vi "Cycle_Diag_Table_Read.vi"(7 "ERD Data In":T3[](array[typedef]) {"ERD Number" format="%.0x"}, 11 "error in (no error)":errorcluster) -> (2 "Cycle Buffer Status":T2, 3 "Diag Cycle String Out":string[][](array[string]), 8 "Cycle  Diag Array Out":T1[](array[typedef]), 15 "error out":errorcluster)   [LabVIEW 2016]
uses:
  Common/LabVIEW GEA2 Toolkit/LabVIEW_GEA2_Toolkit.lvlibp/type defs/ERD Read Data Out.ctl
  type defs/Cycle_Diag_Buffer_Status.ctl
  type defs/Cycle_Diag.ctl
  Common/LabVIEW GEA2 Toolkit/LabVIEW_GEA2_Toolkit.lvlibp
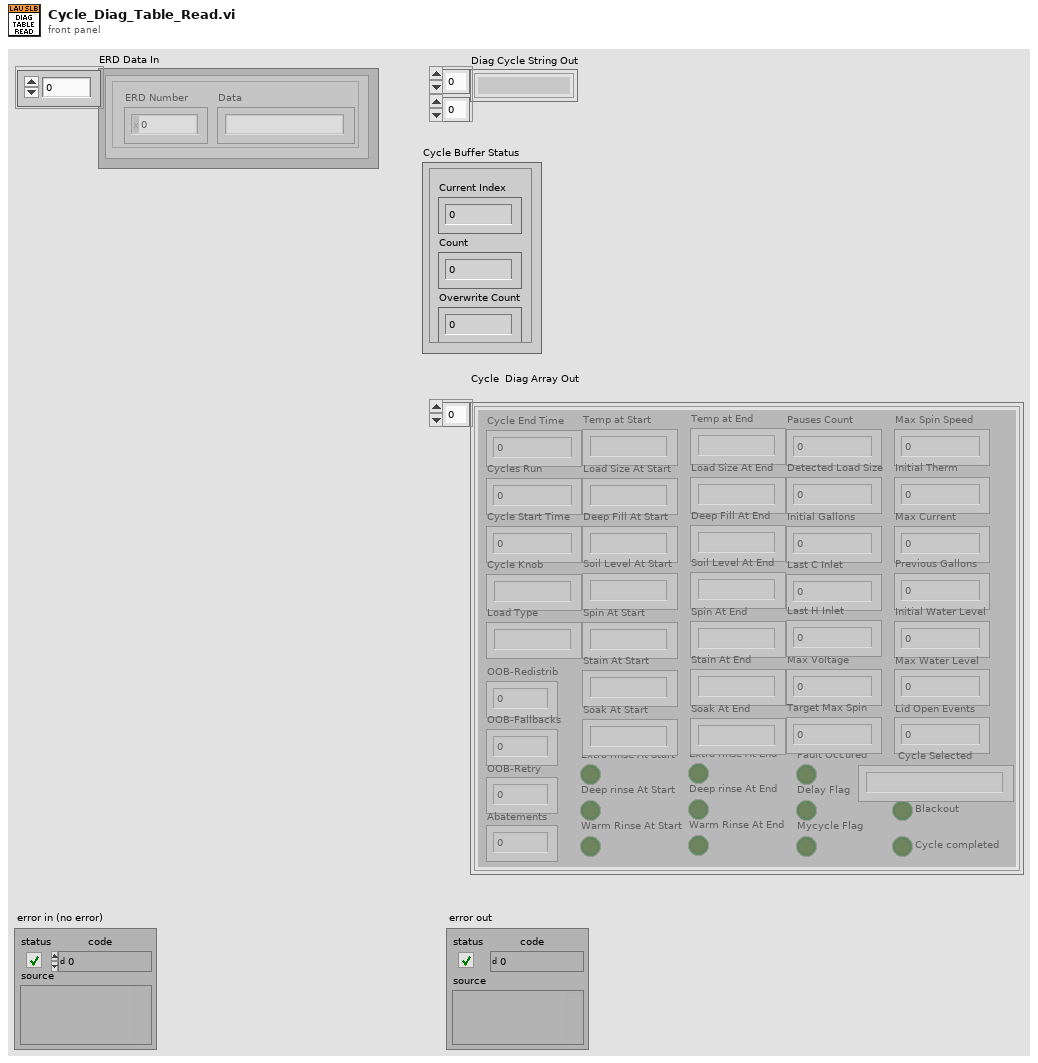
[diagram p1: front panel]
types:
  T1 = typedef "Cycle_Diag.ctl" = cluster{"Cycle End Time":u32, "Cycles Run":u32, "Cycle Start Time":u32, "Cycle Knob":string, "Load Type":string, "OOB-Redistrib":u8, "OOB-Fallbacks":u8, "OOB-Retry":u8, "Temp at Start":string, "Load Size At Start":string, "Deep Fill At Start":string, "Soil Level At Start":string, "Spin At Start":string, "Extra rinse At Start":bool, "Deep rinse At Start":bool, "Stain At Start":string, "Soak At Start":string, "Warm Rinse At Start":bool, "Temp at End":string, "Load Size At End":string, "Deep Fill At End":string, "Soil Level At End":string, "Spin At End":string, "Extra rinse At End":bool, "Deep rinse At End":bool, "Stain At End":string, "Soak At End":string, "Warm Rinse At End":bool, "Pauses Count":u8, "Fault Occured":bool, "Delay Flag":bool, "Mycycle Flag":bool, "Blackout":bool, "Cycle completed":bool, "Detected Load Size":dbl, "Initial Gallons":dbl, "Last C Inlet ":dbl, "Max Voltage":dbl, "Target Max Spin":u16, "Max Spin Speed":u16, "Initial Therm":dbl, "Max Current":dbl, "Previous Gallons":dbl, "Initial Water Level":dbl, "Max Water Level":dbl, "Abatements ":u8, "Lid Open Events":u8, "Cycle Selected":string, "Last H Inlet ":dbl}
  T2 = typedef "Cycle_Diag_Buffer_Status.ctl" = cluster{"Current Index":u16, "Count":u16, "Overwrite Count":u16}
  T3 = typedef "LabVIEW_GEA2_Toolkit.lvlibp/ERD Read Data Out.ctl" = cluster{"ERD Number":u16, "Data":string}
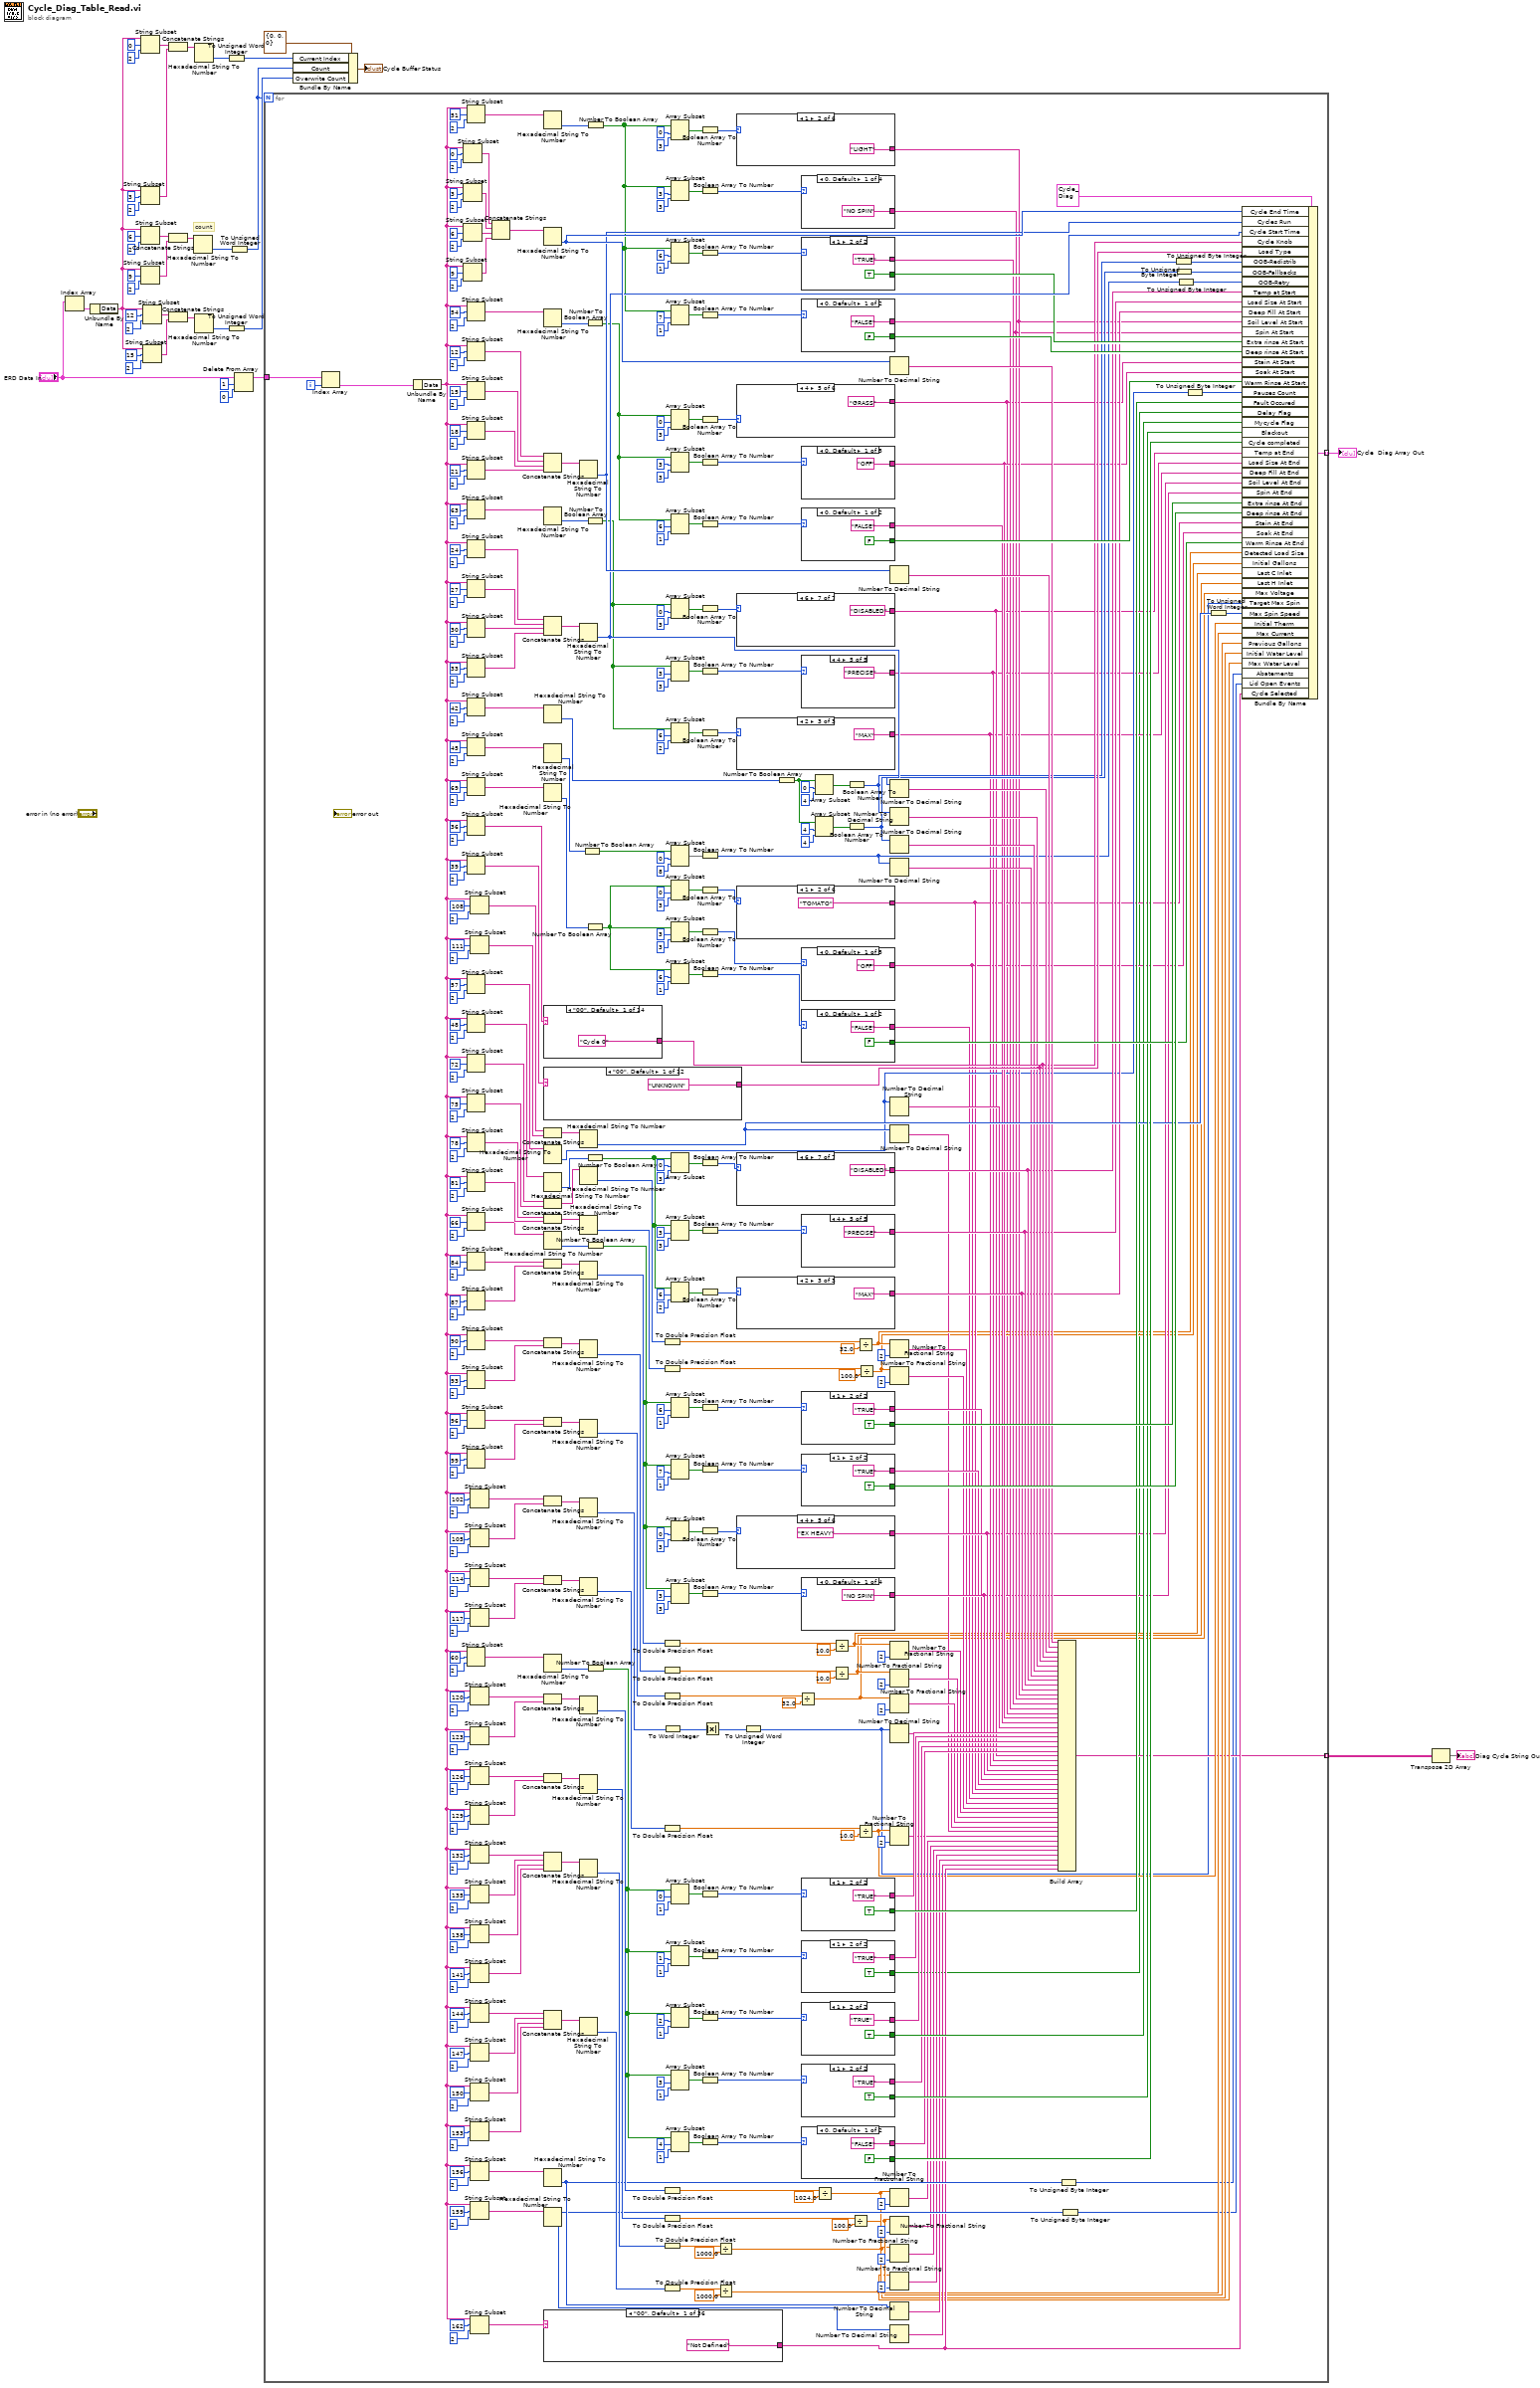
[diagram p0: block diagram]
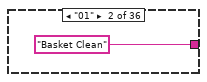
[diagram p2: hidden frame]
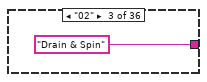
[diagram p3: hidden frame]
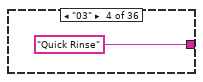
[diagram p4: hidden frame]
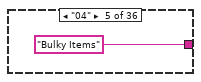
[diagram p5: hidden frame]
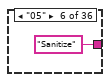
[diagram p6: hidden frame]
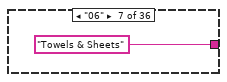
[diagram p7: hidden frame]
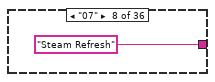
[diagram p8: hidden frame]
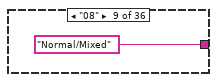
[diagram p9: hidden frame]
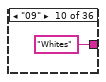
[diagram p10: hidden frame]
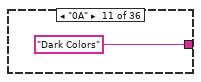
[diagram p11: hidden frame]
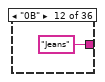
[diagram p12: hidden frame]
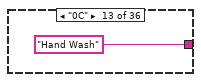
[diagram p13: hidden frame]
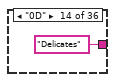
[diagram p14: hidden frame]
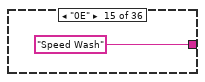
[diagram p15: hidden frame]
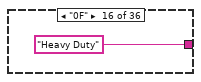
[diagram p16: hidden frame]
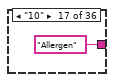
[diagram p17: hidden frame]
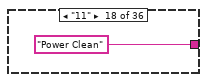
[diagram p18: hidden frame]
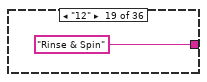
[diagram p19: hidden frame]
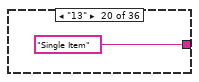
[diagram p20: hidden frame]
diagram:
  # "count"
  n1 = Index Array(array="ERD Data In") -> (element=w31:T3)  [unwired: 1 in]
  n2 = Unbundle By Name(w31) -> ("Data"=w11:string)
  n3 = String Subset(string=w11, offset (0)=0, length (rest)=2 ("length (rest)")) -> (substring=w20:string)
  n4 = String Subset(string=w11, offset (0)=3, length (rest)=2 ("length (rest)")) -> (substring=w21:string)
  n5 = String Subset(string=w11, offset (0)=6, length (rest)=2 ("length (rest)")) -> (substring=w35:string)
  n6 = String Subset(string=w11, offset (0)=9, length (rest)=2 ("length (rest)")) -> (substring=w34:string)
  n7 = String Subset(string=w11, offset (0)=12, length (rest)=2 ("length (rest)")) -> (substring=w22:string)
  n8 = String Subset(string=w11, offset (0)=15, length (rest)=2 ("length (rest)")) -> (substring=w23:string)
  n9 = Concatenate Strings(w20, w21) -> (w24:string)
  n10 = Concatenate Strings(w35, w34) -> (w33:string)
  n11 = Concatenate Strings(w22, w23) -> (w25:string)
  n12 = Hexadecimal String To Number(string=w33) -> (number=w32:u32)  [unwired: 2 in, 1 out]
  n13 = Hexadecimal String To Number(string=w24) -> (number=w26:u32)  [unwired: 2 in, 1 out]
  n14 = Hexadecimal String To Number(string=w25) -> (number=w27:u32)  [unwired: 2 in, 1 out]
  n15 = To Unsigned Word Integer(number=w26) -> (unsigned 16bit integer=w28:u16)
  n16 = To Unsigned Word Integer(number=w27) -> (unsigned 16bit integer=w29:u16)
  n17 = To Unsigned Word Integer(number=w32) -> (unsigned 16bit integer=w10:u16)
  n18 = Delete From Array(array="ERD Data In", length=1, index=0) -> (array with subset deleted=w7:T3[])  [unwired: 1 out]
  n19 = for {
    N: w10 -> [_]
    tunnel: w7 -> [w237]
    tunnel: [w233] -> w3 mode=indexing
    tunnel: [w170] -> w2 mode=indexing
    i -> [w236]
    n20 = Index Array(array=w237, index=w236) -> (element=w235:T3)
    n21 = Unbundle By Name(w235) -> ("Data"=w234:string)
    n22 = String Subset(string=w234, offset (0)=0, length (rest)=2 ("length (rest)")) -> (substring=w451:string)
    n23 = String Subset(string=w234, offset (0)=3, length (rest)=2 ("length (rest)")) -> (substring=w450:string)
    n24 = String Subset(string=w234, offset (0)=6, length (rest)=2 ("length (rest)")) -> (substring=w449:string)
    n25 = String Subset(string=w234, offset (0)=9, length (rest)=2 ("length (rest)")) -> (substring=w448:string)
    n26 = String Subset(string=w234, offset (0)=51, length (rest)=2 ("length (rest)")) -> (substring=w148:string)
    n27 = String Subset(string=w234, offset (0)=54, length (rest)=2 ("length (rest)")) -> (substring=w132:string)
    n28 = String Subset(string=w234, offset (0)=12, length (rest)=2 ("length (rest)")) -> (substring=w445:string)
    n29 = String Subset(string=w234, offset (0)=15, length (rest)=2 ("length (rest)")) -> (substring=w444:string)
    n30 = String Subset(string=w234, offset (0)=18, length (rest)=2 ("length (rest)")) -> (substring=w443:string)
    n31 = String Subset(string=w234, offset (0)=21, length (rest)=2 ("length (rest)")) -> (substring=w442:string)
    n32 = String Subset(string=w234, offset (0)=63, length (rest)=2 ("length (rest)")) -> (substring=w119:string)
    n33 = String Subset(string=w234, offset (0)=24, length (rest)=2 ("length (rest)")) -> (substring=w439:string)
    n34 = String Subset(string=w234, offset (0)=27, length (rest)=2 ("length (rest)")) -> (substring=w438:string)
    n35 = String Subset(string=w234, offset (0)=30, length (rest)=2 ("length (rest)")) -> (substring=w437:string)
    n36 = String Subset(string=w234, offset (0)=33, length (rest)=2 ("length (rest)")) -> (substring=w436:string)
    n37 = String Subset(string=w234, offset (0)=42, length (rest)=2 ("length (rest)")) -> (substring=w88:string)
    n38 = String Subset(string=w234, offset (0)=45, length (rest)=2 ("length (rest)")) -> (substring=w79:string)
    n39 = String Subset(string=w234, offset (0)=69, length (rest)=2 ("length (rest)")) -> (substring=w92:string)
    n40 = String Subset(string=w234, offset (0)=36, length (rest)=2 ("length (rest)")) -> (substring=w433:string)
    n41 = String Subset(string=w234, offset (0)=39, length (rest)=2 ("length (rest)")) -> (substring=w432:string)
    n42 = String Subset(string=w234, offset (0)=57, length (rest)=2 ("length (rest)")) -> (substring=w390:string)
    n43 = String Subset(string=w234, offset (0)=48, length (rest)=2 ("length (rest)")) -> (substring=w167:string)
    n44 = String Subset(string=w234, offset (0)=72, length (rest)=2 ("length (rest)")) -> (substring=w374:string)
    n45 = String Subset(string=w234, offset (0)=75 ("offset"), length (rest)=u32 2 ("default (0 U32)")) -> (substring=w371:string)
    n46 = String Subset(string=w234, offset (0)=78, length (rest)=2 ("length (rest)")) -> (substring=w366:string)
    n47 = String Subset(string=w234, offset (0)=81, length (rest)=2 ("length (rest)")) -> (substring=w365:string)
    n48 = String Subset(string=w234, offset (0)=66, length (rest)=2 ("length (rest)")) -> (substring=w105:string)
    n49 = String Subset(string=w234, offset (0)=84, length (rest)=2 ("length (rest)")) -> (substring=w355:string)
    n50 = String Subset(string=w234, offset (0)=87, length (rest)=2 ("length (rest)")) -> (substring=w354:string)
    n51 = String Subset(string=w234, offset (0)=90, length (rest)=2 ("length (rest)")) -> (substring=w349:string)
    n52 = String Subset(string=w234, offset (0)=93, length (rest)=2 ("length (rest)")) -> (substring=w348:string)
    n53 = String Subset(string=w234, offset (0)=96, length (rest)=2 ("length (rest)")) -> (substring=w339:string)
    n54 = String Subset(string=w234, offset (0)=99, length (rest)=2 ("length (rest)")) -> (substring=w338:string)
    n55 = String Subset(string=w234, offset (0)=60, length (rest)=2 ("length (rest)")) -> (substring=w389:string)
    n56 = String Subset(string=w234, offset (0)=108, length (rest)=2 ("length (rest)")) -> (substring=w326:string)
    n57 = String Subset(string=w234, offset (0)=111, length (rest)=2 ("length (rest)")) -> (substring=w325:string)
    n58 = String Subset(string=w234, offset (0)=102, length (rest)=2 ("length (rest)")) -> (substring=w329:string)
    n59 = String Subset(string=w234, offset (0)=105, length (rest)=2 ("length (rest)")) -> (substring=w328:string)
    n60 = String Subset(string=w234, offset (0)=114, length (rest)=2 ("length (rest)")) -> (substring=w314:string)
    n61 = String Subset(string=w234, offset (0)=117, length (rest)=2 ("length (rest)")) -> (substring=w313:string)
    n62 = String Subset(string=w234, offset (0)=120, length (rest)=2 ("length (rest)")) -> (substring=w304:string)
    n63 = String Subset(string=w234, offset (0)=123, length (rest)=2 ("length (rest)")) -> (substring=w303:string)
    n64 = String Subset(string=w234, offset (0)=126, length (rest)=2 ("length (rest)")) -> (substring=w294:string)
    n65 = String Subset(string=w234, offset (0)=129, length (rest)=2 ("length (rest)")) -> (substring=w293:string)
    n66 = String Subset(string=w234, offset (0)=132, length (rest)=2 ("length (rest)")) -> (substring=w284:string)
    n67 = String Subset(string=w234, offset (0)=135, length (rest)=2 ("length (rest)")) -> (substring=w283:string)
    n68 = String Subset(string=w234, offset (0)=138, length (rest)=2 ("length (rest)")) -> (substring=w253:string)
    n69 = String Subset(string=w234, offset (0)=141, length (rest)=2 ("length (rest)")) -> (substring=w252:string)
    n70 = String Subset(string=w234, offset (0)=144, length (rest)=2 ("length (rest)")) -> (substring=w278:string)
    n71 = String Subset(string=w234, offset (0)=147, length (rest)=2 ("length (rest)")) -> (substring=w277:string)
    n72 = String Subset(string=w234, offset (0)=150, length (rest)=2 ("length (rest)")) -> (substring=w247:string)
    n73 = String Subset(string=w234, offset (0)=153, length (rest)=2 ("length (rest)")) -> (substring=w246:string)
    n74 = String Subset(string=w234, offset (0)=156, length (rest)=2 ("length (rest)")) -> (substring=w258:string)
    n75 = String Subset(string=w234, offset (0)=159, length (rest)=2 ("length (rest)")) -> (substring=w257:string)
    n76 = String Subset(string=w234, offset (0)=162, length (rest)=2 ("length (rest)")) -> (substring=w254:string)
    n77 = Concatenate Strings(w451, w450, w449, w448) -> (w447:string)
    n78 = Hexadecimal String To Number(string=w148) -> (number=w155:u32)  [unwired: 2 in, 1 out]
    n79 = Hexadecimal String To Number(string=w447) -> (number=w446:u32)  [unwired: 2 in, 1 out]
    n80 = Hexadecimal String To Number(string=w132) -> (number=w140:u32)  [unwired: 2 in, 1 out]
    n81 = Concatenate Strings(w445, w444, w443, w442) -> (w441:string)
    n82 = Hexadecimal String To Number(string=w119) -> (number=w127:u32)  [unwired: 2 in, 1 out]
    n83 = Concatenate Strings(w439, w438, w437, w436) -> (w435:string)
    n84 = Hexadecimal String To Number(string=w88) -> (number=w87:u32)  [unwired: 2 in, 1 out]
    n85 = Hexadecimal String To Number(string=w79) -> (number=w78:u32)  [unwired: 2 in, 1 out]
    n86 = Hexadecimal String To Number(string=w92) -> (number=w100:u32)  [unwired: 2 in, 1 out]
    n87 = case shown="\"00\", Default" w433 {
      tunnel: ["Cycle 0" "Cycle 1" "Cycle 2" "Cycle 3" "Cycle 4" "Cycle 5" "Cycle 6" "Cycle 7" "Cycle 8" "Cycle 9" "Cycle 10" "Cycle 11" "Cycle 12" "Cycle 13"] -> w229
      frame "00", Default {
      }
      frame "01" {
      }
      frame "02" {
      }
      frame "03" {
      }
      frame "04" {
      }
      frame "05" {
      }
      frame "06" {
      }
      frame "07" {
      }
      frame "08" {
      }
      frame "09" {
      }
      frame "0A" {
      }
      frame "0B" {
      }
      frame "0C" {
      }
      frame "0D" {
      }
    }
    n88 = case shown="\"00\", Default" w432 {
      tunnel: ["UNKNOWN" "COTTON" "SYNTHETIC" "MIXED" "WET" "LOW FLOW" "SMALL" "MEDIUM" "LARGE" "SUPER" "SUPER PLUS" "MAX"] -> w228
      frame "00", Default {
      }
      frame "01" {
      }
      frame "02" {
      }
      frame "03" {
      }
      frame "04" {
      }
      frame "05" {
      }
      frame "06" {
      }
      frame "07" {
      }
      frame "08" {
      }
      frame "09" {
      }
      frame "0A" {
      }
      frame "0B" {
      }
    }
    n89 = Concatenate Strings(w326, w325) -> (w324:string)
    n90 = Hexadecimal String To Number(string=w390) -> (number=w212:u32)  [unwired: 2 in, 1 out]
    n91 = Hexadecimal String To Number(string=w167) -> (number=w166:u32)  [unwired: 2 in, 1 out]
    n92 = Concatenate Strings(w374, w371) -> (w370:string)
    n93 = Concatenate Strings(w366, w365) -> (w364:string)
    n94 = Hexadecimal String To Number(string=w105) -> (number=w115:u32)  [unwired: 2 in, 1 out]
    n95 = Concatenate Strings(w355, w354) -> (w353:string)
    n96 = Concatenate Strings(w349, w348) -> (w347:string)
    n97 = Concatenate Strings(w339, w338) -> (w337:string)
    n98 = Concatenate Strings(w329, w328) -> (w327:string)
    n99 = Concatenate Strings(w314, w313) -> (w312:string)
    n100 = Hexadecimal String To Number(string=w389) -> (number=w388:u32)  [unwired: 2 in, 1 out]
    n101 = Concatenate Strings(w304, w303) -> (w302:string)
    n102 = Concatenate Strings(w294, w293) -> (w292:string)
    n103 = Concatenate Strings(w284, w283, w253, w252) -> (w282:string)
    n104 = Concatenate Strings(w278, w277, w247, w246) -> (w276:string)
    n105 = Hexadecimal String To Number(string=w258) -> (number=w256:u32)  [unwired: 2 in, 1 out]
    n106 = Hexadecimal String To Number(string=w257) -> (number=w255:u32)  [unwired: 2 in, 1 out]
    n107 = case shown="\"00\", Default" w254 {
      tunnel: ["Not Defined" "Basket Clean" "Drain & Spin" "Quick Rinse" "Bulky Items" "Sanitize" "Towels & Sheets" "Steam Refresh" "Normal/Mixed" "Whites" "Dark Colors" "Jeans" "Hand Wash" "Delicates" "Speed Wash" "Heavy Duty" "Allergen" "Power Clean" "Rinse & Spin" "Single Item" "Colors" "Cold Wash" "Cottons" "Easy Care" "Active Wear" "Timed Dry" "Dewrinkle" "Air Fluff" "Steam Refresh" "Steam Dewrinkle" "Speed Dry" "Mixed" "Quick Dry" "Casuals" "Warm Up" "Energy Saver"] -> w179
      frame "00", Default {
      }
      frame "01" {
      }
      frame "02" {
      }
      frame "03" {
      }
      frame "04" {
      }
      frame "05" {
      }
      frame "06" {
      }
      frame "07" {
      }
      frame "08" {
      }
      frame "09" {
      }
      frame "0A" {
      }
      frame "0B" {
      }
      frame "0C" {
      }
      frame "0D" {
      }
      frame "0E" {
      }
      frame "0F" {
      }
      frame "10" {
      }
      frame "11" {
      }
      frame "12" {
      }
      frame "13" {
      }
      frame "14" {
      }
      frame "15" {
      }
      frame "80" {
      }
      frame "81" {
      }
      frame "82" {
      }
      frame "83" {
      }
      frame "84" {
      }
      frame "85" {
      }
      frame "86" {
      }
      frame "87" {
      }
      frame "88" {
      }
      frame "89" {
      }
      frame "8A" {
      }
      frame "8B" {
      }
      frame "8C" {
      }
      frame "8D" {
      }
    }
    n108 = Hexadecimal String To Number(string=w441) -> (number=w440:u32)  [unwired: 2 in, 1 out]
    n109 = Hexadecimal String To Number(string=w435) -> (number=w434:u32)  [unwired: 2 in, 1 out]
    n110 = Hexadecimal String To Number(string=w324) -> (number=w323:u32)  [unwired: 2 in, 1 out]
    n111 = Hexadecimal String To Number(string=w370) -> (number=w377:u32)  [unwired: 2 in, 1 out]
    n112 = Hexadecimal String To Number(string=w364) -> (number=w363:u32)  [unwired: 2 in, 1 out]
    n113 = Hexadecimal String To Number(string=w353) -> (number=w352:u32)  [unwired: 2 in, 1 out]
    n114 = Hexadecimal String To Number(string=w347) -> (number=w346:u32)  [unwired: 2 in, 1 out]
    n115 = Hexadecimal String To Number(string=w337) -> (number=w336:u32)  [unwired: 2 in, 1 out]
    n116 = Hexadecimal String To Number(string=w327) -> (number=w239:u32)  [unwired: 2 in, 1 out]
    n117 = Hexadecimal String To Number(string=w312) -> (number=w311:u32)  [unwired: 2 in, 1 out]
    n118 = Hexadecimal String To Number(string=w302) -> (number=w301:u32)  [unwired: 2 in, 1 out]
    n119 = Hexadecimal String To Number(string=w292) -> (number=w291:u32)  [unwired: 2 in, 1 out]
    n120 = Hexadecimal String To Number(string=w282) -> (number=w281:u32)  [unwired: 2 in, 1 out]
    n121 = Hexadecimal String To Number(string=w276) -> (number=w275:u32)  [unwired: 2 in, 1 out]
    n122 = Number To Boolean Array(number=w78) -> (Boolean array=w77:bool[])
    n123 = Number To Boolean Array(number=w140) -> (Boolean array=w139:bool[])
    n124 = Number To Boolean Array(number=w127) -> (Boolean array=w126:bool[])
    n125 = Number To Boolean Array(number=w100) -> (Boolean array=w99:bool[])
    n126 = Number To Boolean Array(number=w166) -> (Boolean array=w165:bool[])
    n127 = Number To Boolean Array(number=w155) -> (Boolean array=w147:bool[])
    n128 = Number To Boolean Array(number=w115) -> (Boolean array=w108:bool[])
    n129 = Number To Boolean Array(number=w388) -> (Boolean array=w63:bool[])
    n130 = To Double Precision Float(number=w377) -> (double precision float=w376:dbl)
    n131 = To Double Precision Float(number=w363) -> (double precision float=w362:dbl)
    n132 = To Double Precision Float(number=w352) -> (double precision float=w351:dbl)
    n133 = To Double Precision Float(number=w346) -> (double precision float=w345:dbl)
    n134 = To Double Precision Float(number=w336) -> (double precision float=w335:dbl)
    n135 = To Word Integer(number=w239) -> (16bit integer=w241:i16)
    n136 = To Double Precision Float(number=w311) -> (double precision float=w310:dbl)
    n137 = To Double Precision Float(number=w301) -> (double precision float=w300:dbl)
    n138 = To Double Precision Float(number=w291) -> (double precision float=w290:dbl)
    n139 = To Double Precision Float(number=w281) -> (double precision float=w280:dbl)
    n140 = To Double Precision Float(number=w275) -> (double precision float=w274:dbl)
    n141 = Array Subset(array=w147, index=0, length=3) -> (w144:bool[])
    n142 = Array Subset(array=w147, index=3, length=3) -> (w143:bool[])
    n143 = Array Subset(array=w147, index=6, length=1) -> (w142:bool[])
    n144 = Array Subset(array=w147, index=7, length=1) -> (w141:bool[])
    n145 = Array Subset(array=w139, index=0, length=3) -> (w130:bool[])
    n146 = Array Subset(array=w139, index=3, length=3) -> (w129:bool[])
    n147 = Array Subset(array=w139, index=6, length=1) -> (w128:bool[])
    n148 = Array Subset(array=w126, index=0, length=3) -> (w118:bool[])
    n149 = Array Subset(array=w126, index=3, length=3) -> (w117:bool[])
    n150 = Array Subset(array=w126, index=6, length=2) -> (w116:bool[])
    n151 = Array Subset(array=w77, index=0, length=8) -> (w74:bool[])
    n152 = Array Subset(array=w99, index=0, length=3) -> (w91:bool[])
    n153 = Array Subset(array=w99, index=3, length=3) -> (w90:bool[])
    n154 = Array Subset(array=w99, index=6, length=1) -> (w89:bool[])
    n155 = Array Subset(array=w165, index=0, length=3) -> (w158:bool[])
    n156 = Array Subset(array=w165, index=3, length=3) -> (w157:bool[])
    n157 = Array Subset(array=w165, index=6, length=2) -> (w156:bool[])
    n158 = Array Subset(array=w108, index=6, length=1) -> (w102:bool[])
    n159 = Array Subset(array=w108, index=7, length=1) -> (w101:bool[])
    n160 = Array Subset(array=w108, index=0, length=3) -> (w104:bool[])
    n161 = Array Subset(array=w108, index=3, length=3) -> (w103:bool[])
    n162 = Array Subset(array=w63, index=0, length=1) -> (w62:bool[])
    n163 = Array Subset(array=w63, index=1, length=1) -> (w60:bool[])
    n164 = Array Subset(array=w63, index=2, length=1) -> (w59:bool[])
    n165 = Array Subset(array=w63, index=3, length=1) -> (w58:bool[])
    n166 = Array Subset(array=w63, index=4, length=1) -> (w57:bool[])
    n167 = Boolean Array To Number(Boolean array=w144) -> (number=w423:u32)
    n168 = Boolean Array To Number(Boolean array=w143) -> (number=w422:u32)
    n169 = Boolean Array To Number(Boolean array=w142) -> (number=w421:u32)
    n170 = Boolean Array To Number(Boolean array=w141) -> (number=w420:u32)
    n171 = Boolean Array To Number(Boolean array=w130) -> (number=w417:u32)
    n172 = Boolean Array To Number(Boolean array=w129) -> (number=w416:u32)
    n173 = Boolean Array To Number(Boolean array=w128) -> (number=w415:u32)
    n174 = Boolean Array To Number(Boolean array=w118) -> (number=w407:u32)
    n175 = Boolean Array To Number(Boolean array=w117) -> (number=w406:u32)
    n176 = Boolean Array To Number(Boolean array=w116) -> (number=w405:u32)
    n177 = Boolean Array To Number(Boolean array=w74) -> (number=w222:u32)
    n178 = Boolean Array To Number(Boolean array=w91) -> (number=w400:u32)
    n179 = Boolean Array To Number(Boolean array=w90) -> (number=w399:u32)
    n180 = Boolean Array To Number(Boolean array=w89) -> (number=w398:u32)
    n181 = Boolean Array To Number(Boolean array=w158) -> (number=w238:u32)
    n182 = Boolean Array To Number(Boolean array=w157) -> (number=w425:u32)
    n183 = Boolean Array To Number(Boolean array=w156) -> (number=w424:u32)
    n184 = Boolean Array To Number(Boolean array=w102) -> (number=w402:u32)
    n185 = Boolean Array To Number(Boolean array=w101) -> (number=w401:u32)
    n186 = Boolean Array To Number(Boolean array=w104) -> (number=w404:u32)
    n187 = Boolean Array To Number(Boolean array=w103) -> (number=w403:u32)
    n188 = Boolean Array To Number(Boolean array=w62) -> (number=w387:u32)
    n189 = Boolean Array To Number(Boolean array=w60) -> (number=w386:u32)
    n190 = Boolean Array To Number(Boolean array=w59) -> (number=w385:u32)
    n191 = Boolean Array To Number(Boolean array=w58) -> (number=w384:u32)
    n192 = Boolean Array To Number(Boolean array=w57) -> (number=w383:u32)
    n193 = Absolute Value(x=w241) -> (abs(x)=w240:i16)
    n194 = Divide(x=w280, y=1000.0) -> (x/y=w172:dbl)
    n195 = Divide(x=w274, y=1000.0) -> (x/y=w171:dbl)
    n196 = case shown="1" w423 {
      tunnel: ["EXTRA LIGHT" "LIGHT" "NORMAL" "HEAVY" "EX HEAVY" "DISABLED"] -> w218
      frame 0, Default {
      }
      frame 1 {
      }
      frame 2 {
      }
      frame 3 {
      }
      frame 4 {
      }
      frame 5 {
      }
    }
    n197 = case shown="4" w417 {
      tunnel: ["OFF" "TOMATO" "WINE" "BLOOD" "GRASS" "DIRT"] -> w131
      frame 0, Default {
      }
      frame 1 {
      }
      frame 2 {
      }
      frame 3 {
      }
      frame 4 {
      }
      frame 5 {
      }
    }
    n198 = case shown="6" w407 {
      tunnel: ["TAP COLD" "COLD" "COOL" "COLORS" "WARM" "HOT" "DISABLED"] -> w204
      frame 0, Default {
      }
      frame 1 {
      }
      frame 2 {
      }
      frame 3 {
      }
      frame 4 {
      }
      frame 5 {
      }
      frame 6 {
      }
    }
    n199 = case shown="2" w405 {
      tunnel: ["OFF" "INCREMENTAL" "MAX"] -> w202
      frame 0, Default {
      }
      frame 1 {
      }
      frame 2 {
      }
    }
    n200 = case shown="1" w400 {
      tunnel: ["OFF" "TOMATO" "WINE" "BLOOD" "GRASS" "DIRT"] -> w197
      frame 0, Default {
      }
      frame 1 {
      }
      frame 2 {
      }
      frame 3 {
      }
      frame 4 {
      }
      frame 5 {
      }
    }
    n201 = case shown="6" w238 {
      tunnel: ["TAP COLD" "COLD" "COOL" "COLORS" "WARM" "HOT" "DISABLED"] -> w221
      frame 0, Default {
      }
      frame 1 {
      }
      frame 2 {
      }
      frame 3 {
      }
      frame 4 {
      }
      frame 5 {
      }
      frame 6 {
      }
    }
    n202 = case shown="2" w424 {
      tunnel: ["OFF" "INCREMENTAL" "MAX"] -> w219
      frame 0, Default {
      }
      frame 1 {
      }
      frame 2 {
      }
    }
    n203 = case shown="4" w404 {
      tunnel: ["EXTRA LIGHT" "LIGHT" "NORMAL" "HEAVY" "EX HEAVY" "DISABLED"] -> w201
      frame 0, Default {
      }
      frame 1 {
      }
      frame 2 {
      }
      frame 3 {
      }
      frame 4 {
      }
      frame 5 {
      }
    }
    n204 = To Unsigned Word Integer(number=w240) -> (unsigned 16bit integer=w46:u16)
    n205 = Number To Boolean Array(number=w87) -> (Boolean array=w82:bool[])
    n206 = Divide(x=w335, y=32.0) -> (x/y=w176:dbl)
    n207 = case shown="0, Default" w422 {
      tunnel: ["NO SPIN" "NORMAL" "MORE" "MAX"] -> w217
      frame 0, Default {
      }
      frame 1 {
      }
      frame 2 {
      }
      frame 3 {
      }
    }
    n208 = case shown="1" w421 {
      tunnel: [FALSE TRUE] -> w419
      tunnel: ["FALSE" "TRUE"] -> w216
      frame 0, Default {
      }
      frame 1 {
      }
    }
    n209 = case shown="0, Default" w420 {
      tunnel: [FALSE TRUE] -> w418
      tunnel: ["FALSE" "TRUE"] -> w215
      frame 0, Default {
      }
      frame 1 {
      }
    }
    n210 = case shown="0, Default" w416 {
      tunnel: ["OFF" "15 MIN" "30 MIN" "60 MIN" "2 HOURS"] -> w214
      frame 0, Default {
      }
      frame 1 {
      }
      frame 2 {
      }
      frame 3 {
      }
      frame 4 {
      }
    }
    n211 = case shown="0, Default" w415 {
      tunnel: [FALSE TRUE] -> w414
      tunnel: ["FALSE" "TRUE"] -> w213
      frame 0, Default {
      }
      frame 1 {
      }
    }
    n212 = case shown="4" w406 {
      tunnel: ["SMALL" "MEDIUM" "LARGE" "SUPER" "PRECISE"] -> w203
      frame 0, Default {
      }
      frame 1 {
      }
      frame 2 {
      }
      frame 3 {
      }
      frame 4 {
      }
    }
    n213 = case shown="0, Default" w399 {
      tunnel: ["OFF" "15 MIN" "30 MIN" "60 MIN" "2 HOURS"] -> w196
      frame 0, Default {
      }
      frame 1 {
      }
      frame 2 {
      }
      frame 3 {
      }
      frame 4 {
      }
    }
    n214 = case shown="0, Default" w398 {
      tunnel: [FALSE TRUE] -> w395
      tunnel: ["FALSE" "TRUE"] -> w195
      frame 0, Default {
      }
      frame 1 {
      }
    }
    n215 = case shown="4" w425 {
      tunnel: ["SMALL" "MEDIUM" "LARGE" "SUPER" "PRECISE"] -> w220
      frame 0, Default {
      }
      frame 1 {
      }
      frame 2 {
      }
      frame 3 {
      }
      frame 4 {
      }
    }
    n216 = case shown="1" w402 {
      tunnel: [FALSE TRUE] -> w397
      tunnel: ["FALSE" "TRUE"] -> w199
      frame 0, Default {
      }
      frame 1 {
      }
    }
    n217 = case shown="1" w401 {
      tunnel: [FALSE TRUE] -> w396
      tunnel: ["FALSE" "TRUE"] -> w198
      frame 0, Default {
      }
      frame 1 {
      }
    }
    n218 = case shown="0, Default" w403 {
      tunnel: ["NO SPIN" "NORMAL" "MORE" "MAX"] -> w200
      frame 0, Default {
      }
      frame 1 {
      }
      frame 2 {
      }
      frame 3 {
      }
    }
    n219 = case shown="1" w387 {
      tunnel: [FALSE TRUE] -> w382
      tunnel: ["FALSE" "TRUE"] -> w209
      frame 0, Default {
      }
      frame 1 {
      }
    }
    n220 = case shown="1" w386 {
      tunnel: [FALSE TRUE] -> w61
      tunnel: ["FALSE" "TRUE"] -> w208
      frame 0, Default {
      }
      frame 1 {
      }
    }
    n221 = case shown="1" w385 {
      tunnel: [FALSE TRUE] -> w210
      tunnel: ["FALSE" "TRUE"] -> w207
      frame 0, Default {
      }
      frame 1 {
      }
    }
    n222 = case shown="1" w384 {
      tunnel: [FALSE TRUE] -> w381
      tunnel: ["FALSE" "TRUE"] -> w206
      frame 0, Default {
      }
      frame 1 {
      }
    }
    n223 = case shown="0, Default" w383 {
      tunnel: [FALSE TRUE] -> w380
      tunnel: ["FALSE" "TRUE"] -> w205
      frame 0, Default {
      }
      frame 1 {
      }
    }
    n224 = Array Subset(array=w82, index=0, length=4) -> (w81:bool[])
    n225 = Array Subset(array=w82, index=4, length=4) -> (w80:bool[])
    n226 = Divide(x=w300, y=1024.0) -> (x/y=w174:dbl)
    n227 = Divide(x=w351, y=10.0) -> (x/y=w178:dbl)
    n228 = Divide(x=w345, y=10.0) -> (x/y=w177:dbl)
    n229 = Boolean Array To Number(Boolean array=w81) -> (number=w227:u32)
    n230 = Boolean Array To Number(Boolean array=w80) -> (number=w225:u32)
    n231 = Divide(x=w290, y=100.0) -> (x/y=w173:dbl)
    n232 = Divide(x=w376, y=32.0) -> (x/y=w194:dbl)
    n233 = Divide(x=w310, y=10.0) -> (x/y=w175:dbl)
    n234 = Divide(x=w362, y=100.0) -> (x/y=w169:dbl)
    n235 = Number To Decimal String(number=w446) -> (decimal integer string=w232:string)  [unwired: 1 in]
    n236 = Number To Decimal String(number=w440) -> (decimal integer string=w231:string)  [unwired: 1 in]
    n237 = Number To Decimal String(number=w434) -> (decimal integer string=w230:string)  [unwired: 1 in]
    n238 = Number To Decimal String(number=w227) -> (decimal integer string=w226:string)  [unwired: 1 in]
    n239 = Number To Decimal String(number=w225) -> (decimal integer string=w224:string)  [unwired: 1 in]
    n240 = Number To Decimal String(number=w222) -> (decimal integer string=w223:string)  [unwired: 1 in]
    n241 = Number To Decimal String(number=w212) -> (decimal integer string=w211:string)  [unwired: 1 in]
    n242 = Number To Decimal String(number=w323) -> (decimal integer string=w187:string)  [unwired: 1 in]
    n243 = Number To Fractional String(number=w194, precision (6)=i16 2) -> (F-format string=w193:string)  [unwired: 2 in]
    n244 = Number To Fractional String(number=w169, precision (6)=i16 2) -> (F-format string=w192:string)  [unwired: 2 in]
    n245 = Number To Fractional String(number=w178, precision (6)=i16 2) -> (F-format string=w191:string)  [unwired: 2 in]
    n246 = Number To Fractional String(number=w177, precision (6)=i16 2) -> (F-format string=w190:string)  [unwired: 2 in]
    n247 = Number To Fractional String(number=w176, precision (6)=i16 2) -> (F-format string=w189:string)  [unwired: 2 in]
    n248 = Number To Decimal String(number=w46) -> (decimal integer string=w188:string)  [unwired: 1 in]
    n249 = Number To Fractional String(number=w175, precision (6)=i16 2) -> (F-format string=w186:string)  [unwired: 2 in]
    n250 = Number To Fractional String(number=w174, precision (6)=i16 2) -> (F-format string=w185:string)  [unwired: 2 in]
    n251 = Number To Fractional String(number=w173, precision (6)=i16 2) -> (F-format string=w184:string)  [unwired: 2 in]
    n252 = Number To Fractional String(number=w172, precision (6)=i16 2) -> (F-format string=w183:string)  [unwired: 2 in]
    n253 = Number To Fractional String(number=w171, precision (6)=i16 2) -> (F-format string=w182:string)  [unwired: 2 in]
    n254 = Number To Decimal String(number=w256) -> (decimal integer string=w181:string)  [unwired: 1 in]
    n255 = Number To Decimal String(number=w255) -> (decimal integer string=w180:string)  [unwired: 1 in]
    n256 = Build Array(w232, w231, w230, w229, w228, w226, w224, w223, w221, w220, w219, w218, w217, w216, w215, w131, w214, w213, w211, w209, w208, w207, w206, w205, w204, w203, w202, w201, w200, w199, w198, w197, w196, w195, w193, w192, w191, w190, w189, w188, w187, w186, w185, w184, w183, w182, w181, w180, w179) -> (w170:string[])
    n257 = To Unsigned Byte Integer(number=w256) -> (unsigned 8bit integer=w45:u8)
    n258 = To Unsigned Byte Integer(number=w255) -> (unsigned 8bit integer=w44:u8)
    n259 = To Unsigned Byte Integer(number=w227) -> (unsigned 8bit integer=w56:u8)
    n260 = To Unsigned Byte Integer(number=w225) -> (unsigned 8bit integer=w55:u8)
    n261 = To Unsigned Byte Integer(number=w222) -> (unsigned 8bit integer=w54:u8)
    n262 = To Unsigned Byte Integer(number=w212) -> (unsigned 8bit integer=w53:u8)
    n263 = To Unsigned Word Integer(number=w323) -> (unsigned 16bit integer=w47:u16)
    n264 = Bundle By Name(cluster=T1 {"Cycle End Time"=0, "Cycles Run"=0, "Cycle Start Time"=0, "Cycle Knob"="", "Load Type"="", "OOB-Redistrib"=0, "OOB-Fallbacks"=0, "OOB-Retry"=0, "Temp at Start"="", "Load Size At Start"="", "Deep Fill At Start"="", "Soil Level At Start"="", "Spin At Start"="", "Extra rinse At Start"=FALSE, "Deep rinse At Start"=FALSE, "Stain At Start"="", "Soak At Start"="", "Warm Rinse At Start"=FALSE, "Temp at End"="", "Load Size At End"="", "Deep Fill At End"="", "Soil Level At End"="", "Spin At End"="", "Extra rinse At End"=FALSE, "Deep rinse At End"=FALSE, "Stain At End"="", "Soak At End"="", "Warm Rinse At End"=FALSE, "Pauses Count"=0, "Fault Occured"=FALSE, "Delay Flag"=FALSE, "Mycycle Flag"=FALSE, "Blackout"=FALSE, "Cycle completed"=FALSE, "Detected Load Size"=0.0, "Initial Gallons"=0.0, "Last C Inlet "=0.0, "Max Voltage"=0.0, "Target Max Spin"=0, "Max Spin Speed"=0, "Initial Therm"=0.0, "Max Current"=0.0, "Previous Gallons"=0.0, "Initial Water Level"=0.0, "Max Water Level"=0.0, "Abatements "=0, "Lid Open Events"=0, "Cycle Selected"="", "Last H Inlet "=0.0} ("Cycle History Diagnostics"), "Cycle End Time"=w446, "Cycles Run"=w440, "Cycle Start Time"=w434, "Cycle Knob"=w229, "Load Type"=w228, "OOB-Redistrib"=w56, "OOB-Fallbacks"=w55, "OOB-Retry"=w54, "Temp at Start"=w221, "Load Size At Start"=w220, "Deep Fill At Start"=w219, "Soil Level At Start"=w218, "Spin At Start"=w217, "Extra rinse At Start"=w419, "Deep rinse At Start"=w418, "Stain At Start"=w131, "Soak At Start"=w214, "Warm Rinse At Start"=w414, "Pauses Count"=w53, "Fault Occured"=w382, "Delay Flag"=w61, "Mycycle Flag"=w210, "Blackout"=w381, "Cycle completed"=w380, "Temp at End"=w204, "Load Size At End"=w203, "Deep Fill At End"=w202, "Soil Level At End"=w201, "Spin At End"=w200, "Extra rinse At End"=w397, "Deep rinse At End"=w396, "Stain At End"=w197, "Soak At End"=w196, "Warm Rinse At End"=w395, "Detected Load Size"=w194, "Initial Gallons"=w169, "Last C Inlet"=w178, "Last H Inlet"=w177, "Max Voltage"=w176, "Target Max Spin"=w46, "Max Spin Speed"=w47, "Initial Therm"=w175, "Max Current"=w174, "Previous Gallons"=w173, "Initial Water Level"=w172, "Max Water Level"=w171, "Abatements"=w45, "Lid Open Events"=w44, "Cycle Selected"=w179) -> (w233:T1)
  }
  "Cycle  Diag Array Out" <- w3
  n265 = Bundle By Name(cluster=T2 {"Current Index"=0, "Count"=0, "Overwrite Count"=0} ("Cycle Buffer Status"), "Current Index"=w28, "Count"=w10, "Overwrite Count"=w29) -> (→"Cycle Buffer Status":T2)
  n266 = Transpose 2D Array(2D array=w2) -> (transposed array=→"Diag Cycle String Out":string[][])
